vi "ColorMixture.vi"() -> ()   [LabVIEW 2013]
panel:
  out "Array 2":dbl[](array[numeric])
  in  "Reflectance spectrum 2":dbl[](array[numeric])
  in  "Reflectance spectrum":dbl[](array[numeric])
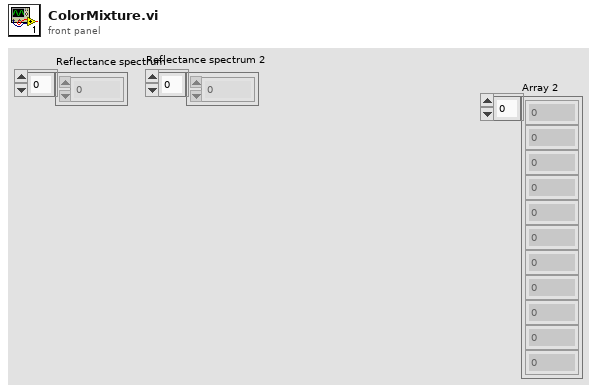
[diagram p1: front panel]
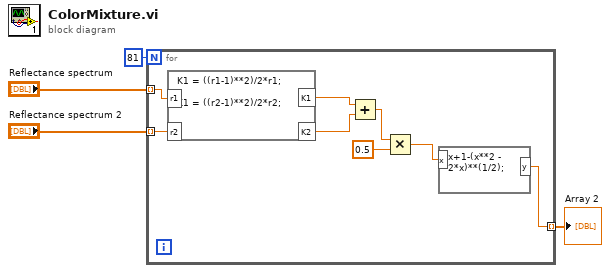
[diagram p0: block diagram]
diagram:
  n1 = for {
    N: 81 -> [_]
    tunnel: "Reflectance spectrum" -> [w9] mode=indexing
    tunnel: "Reflectance spectrum 2" -> [w8] mode=indexing
    tunnel: [w10] -> w1 mode=indexing
    n2 = formula code="K1 = ((r1-1)**2)/2*r1;\n\nK1 = ((r2-1)**2)/2*r2;"("r1"=w9, "r2"=w8) -> ("K1"=w12:dbl, "K2"=w11:dbl)
    n3 = Add(x=w12, y=w11) -> (x+y=w7:dbl)
    n4 = Multiply(x=w7, y=0.5) -> (x*y=w5:dbl)
    n5 = formula code="x+1-(x**2 - 2*x)**(1/2);"("x"=w5) -> ("y"=w10:dbl)
  }
  "Array 2" <- w1
